vi "terminate.vi"(8 "error in (no error)":errorcluster, 11 "ErrorController in":refnum<class "ErrorController.lvclass">) -> (0 "error out":errorcluster, 3 "ErrorController out":refnum<class "ErrorController.lvclass">)   [LabVIEW 2010, in "ErrorController.lvclass"]
doc: "The dynamic dispatch version of this VI terminates the plug-in object by releasing all of its resources."
uses:
  ErrorController.lvclass
  ErrorController.lvclass/ErrorController.ctl
  class_data.vi
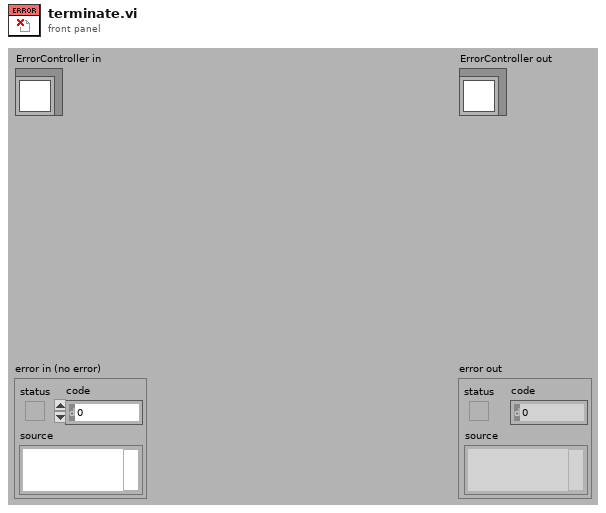
[diagram p1: front panel]
types:
  T1 = typedef "ErrorController.lvclass/queue controller.ctl" = refnum<queue>
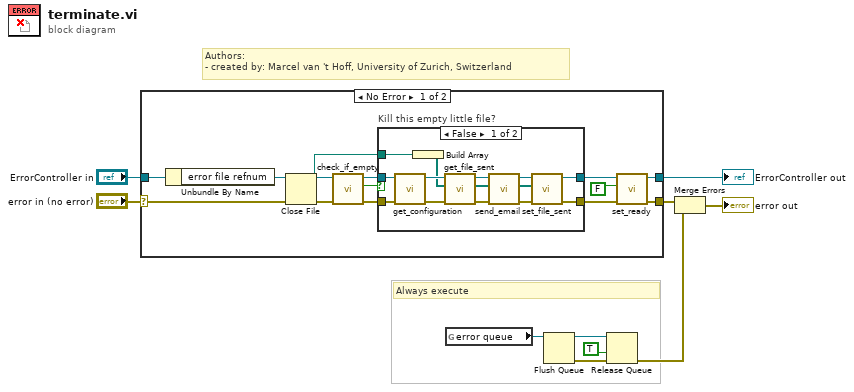
[diagram p0: block diagram]
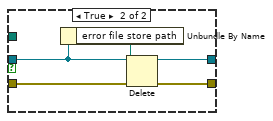
[diagram p2: hidden frame]
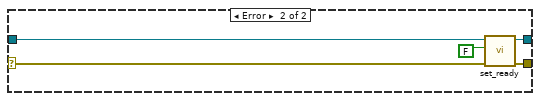
[diagram p3: hidden frame]
diagram:
  # "Authors: \n- created by: Marcel van 't Hoff, University of Zurich, Switzerland"
  # "Always execute"
  n1 = case shown="No Error" "error in (no error)" {
    selector: "error in (no error)" -> [w11 w44]
    tunnel: "ErrorController in" -> [w17 w46]
    tunnel: [w14 w43] -> w7
    tunnel: [w13 w45] -> w9
    frame No Error {
      n2 = Unbundle By Name(w17) -> ("error file refnum"=w19:refnum<file>)
      n3 = Close File(refnum=w19, error in=w11) -> (path=w20:path, error out=w21:errorcluster)
      n4 = call "check_if_empty.vi"("error in (no error)"=w21, "ErrorController"=w17) -> ("error out"=w22:errorcluster, "empty?"=w23:bool, "ErrorController"=w18:refnum<class "ErrorController.lvclass">)  [unwired: 7 in]
      n5 = case "Kill this empty little file?" shown="False" w23 {
        tunnel: [w36 w41] -> w15
        tunnel: w22 -> [w28 w40]
        tunnel: w18 -> [w29 w38]
        tunnel: w20 -> [w25 _]
        tunnel: [w30 w38] -> w16
        frame False {
          n6 = call-dynamic "get_configuration.vi"("error in (no error)"=w28, "ErrorController in"=w29) -> ("error out"=w27:errorcluster, "ErrorController out"=w26:refnum<class "ErrorController.lvclass">)  [unwired: 7 in, 1 out]
          n7 = Build Array(w25) -> (w24:path[])
          n8 = call-dynamic "get_file_sent.vi"("error in (no error)"=w27, "path array in"=w24, "ErrorController in"=w26) -> ("error out"=w32:errorcluster, "path array out"=w34:path[], "ErrorController out"=w33:refnum<class "ErrorController.lvclass">)  [unwired: 6 in]
          n9 = call-dynamic "send_email.vi"("error in (no error)"=w32, "attachments array in"=w34, "ErrorController in"=w33) -> ("error out"=w37:errorcluster, "attachments array out"=w31:path[], "ErrorController out"=w35:refnum<class "ErrorController.lvclass">)  [unwired: 6 in]
          n10 = call-dynamic "set_file_sent.vi"("error in (no error)"=w37, "path array in"=w31, "ErrorController in"=w35) -> ("error out"=w36:errorcluster, "ErrorController out"=w30:refnum<class "ErrorController.lvclass">)  [unwired: 7 in]
        }
        frame True {
          n11 = Unbundle By Name(w38) -> ("error file store path"=w39:path)
          n12 = Delete(path (use dialog)=w39, error in=w40) -> (error out=w41:errorcluster)  [unwired: 3 in, 2 out]
        }
      }
      n13 = call-dynamic "set_ready.vi"("error in (no error)"=w15, "ready?"=FALSE ("Value"), "ErrorController in"=w16) -> ("error out"=w14:errorcluster, "ErrorController out"=w13:refnum<class "ErrorController.lvclass">)  [unwired: 7 in]
    }
    frame Error {
      n14 = call-dynamic "set_ready.vi"("error in (no error)"=w44, "ready?"=FALSE, "ErrorController in"=w46) -> ("error out"=w43:errorcluster, "ErrorController out"=w45:refnum<class "ErrorController.lvclass">)  [unwired: 7 in]
    }
  }
  "ErrorController out" <- w9
  n15 = global read "class_data.vi" "error queue"() -> (w3:T1)
  n16 = Flush Queue(queue=w3) -> (queue out=w2:T1, error out=w1:errorcluster)  [unwired: 1 in, 1 out]
  n17 = Release Queue(queue=w2, force destroy? (F)=TRUE, error in (no error)=w1) -> (error out=w8:errorcluster)  [unwired: 2 out]
  n18 = Merge Errors(w7, w8) -> (→"error out":errorcluster)
